vi "Main FPGA 6-axis Servo 2.vi"() -> ()   [LabVIEW 2014]
uses:
  <vilib>/Motion/MotorControl/_s/nism.encoder.config.ctl
  <vilib>/Motion/MotorControl/_s/nism.encoder.incremental.config.ctl
  <vilib>/Motion/MotorControl/_s/nism.incremental.indexCriteria.ctl
  <vilib>/Motion/MotorControl/_s/nism.pid.gains.fxp.18.ctl
  <vilib>/Motion/MotorControl/_s/nism.pi.v.outputRange.fxp.6.12.ctl
  <vilib>/Motion/MotorControl/_s/nism.mdo.splineData.ctl
  <vilib>/Motion/MotorControl/_s/nism.splineInterpolation.type.ctl
  <vilib>/Motion/SoftMotion/Synchronization/nism.softmotionScan.timerConfig.ctl
  <vilib>/Platform/TimedLoop/XDataNode/timing_clust.ctl
  <vilib>/Platform/TimedLoop/XDataNode/nitl_modes.ctl
  <vilib>/Platform/TimedLoop/XDataNode/wakeup.ctl
  <vilib>/Motion/MotorControl/_s/nism.digitalInputs.portA.ctl
  <vilib>/rvi/Emulation/niFpgaGetClockAttributes.vi
  <vilib>/rvi/Emulation/niFpgaSctlEmulationGetInTimedLoop.vi
  <vilib>/rvi/Emulation/niFpgaEmulationReportErrorSimple.vi
  Global FPGA 6-axis.vi
  <vilib>/Motion/MotorControl/_s/nism.interpretControlRegister.indexed.vi
  <vilib>/rvi/Emulation/niFpgaProcessEmulError.vi
  <vilib>/Motion/MotorControl/_s/nism.mdo.read.encoder.vi
  <vilib>/Motion/MotorControl/_s/nism.mdo.read.positionLoopSyncData.vi
  <vilib>/Motion/MotorControl/_s/nism.mdo.read.splineData.vi
  <vilib>/Motion/MotorControl/_s/nism.generateStatusRegister.indexed.vi
  <vilib>/rvi/eio/common/nirviEmuTemplateMethod_errors.vi
  <vilib>/rvi/Emulation/niFpgaCriticalErrorInLSC.vi
  <vilib>/Motion/MotorControl/_s/nism.splineInterpolation.fxp.3.index.vi
  <vilib>/Motion/MotorControl/_s/nism.pid.simple.fxp.index.2.vi
  <vilib>/Motion/MotorControl/_s/nism.mdo.handler.indexed.vi
  <vilib>/Motion/MotorControl/_s/nism.digitalFilter.indexed.vi
  <vilib>/Motion/MotorControl/_s/nism.interpretDIOControl.portA.multiple.vi
  <vilib>/Motion/MotorControl/_s/nism.generateDIOStatus.portA.indexed.2.vi
  <vilib>/Motion/SoftMotion/Synchronization/nism.rioScan.generateSyncScan.vi
  <vilib>/Motion/MotorControl/_s/nism.incremental.p.2.vi
  <vilib>/eio/EIONode/EIONode.xnode
  <vilib>/Platform/TimedLoop/XDataNode/XDataNode.xnode
  <vilib>/Motion/MotorControl/NI_SoftMotion_MotorControlIP.lvlib
  <vilib>/Platform/TimedLoop/XDataNode/XDNodeRunTimeDep.lvlib
  <vilib>/Motion/SoftMotion/Synchronization/NI_SoftMotion_Synchronization.lvlib
panel:
  in  "Reset Encoder 6":bool caption="reset"
  in  "Reset Encoder 5":bool caption="reset"
  in  "Reset Encoder 4":bool caption="reset"
  in  "Reset Encoder 3":bool caption="reset"
  out "position loop sync":T1
  out "spline":T2 {"spline type" items=["cubic b spline", "catmull-rom spline", "linear"]}
  in  "Reset Encoder 2":bool caption="reset"
  out "Velocity Feedback":i16[](array[numeric])
  out "pos. error":i16[](array[numeric])
  out "pos. error exceeded":bool[](array[boolean])
  in  "calls per sample (vel)":u16=2000 caption="calls per sample"
  in  "Limit Ranges":T4[](array[typedef])=[{"output low"=0.0, "output high"=0.0}, {"output low"=0.0, "output high"=0.0}, {"output low"=0.0, "output high"=0.0}, {"output low"=0.0, "output high"=0.0}, {"output low"=0.0, "output high"=0.0}, {"output low"=0.0, "output high"=0.0}]
  in  "Gains":T5[](array[typedef])=[{"kp"=0.0, "kd"=0.0, "ki"=0.0}, {"kp"=0.0, "kd"=0.0, "ki"=0.0}, {"kp"=0.0, "kd"=0.0, "ki"=0.0}, {"kp"=0.0, "kd"=0.0, "ki"=0.0}, {"kp"=0.0, "kd"=0.0, "ki"=0.0}, {"kp"=0.0, "kd"=0.0, "ki"=0.0}]
  out "AO Check":fxp<+/-,20,5>[](array[numeric])
  in  "AO Manual":fxp<+/-,20,5>[](array[numeric])=[0.0, 0.0, 0.0, 0.0, 0.0, 0.0]
  out "Position Feedback":i32[](array[numeric])
  in  "Reset Encoder 1":bool caption="reset"
  out "corrected period":u16
  in  "AO Disabled?":bool
  out "PID loop time (ticks)":u32
  in  "AO Override?":bool
  in  "position error limit":i16=10000
  in  "Encoder filter value (us) Manual":u16=10
  out "encoder config":T6
  out "Home Limits":bool[](array[boolean])
  out "Fwd Limits":bool[](array[boolean])
  out "Rev Limits":bool[](array[boolean])
  out "Drive Enable":bool[](array[boolean])
  in  "Enable value":bool
  in  "Drive Enable override?":bool
  in  "Sync Value":bool
  in  "Sync Enable override?":bool
  out "Sync is Fault":bool
  out "Sync is Locked":bool
  # "Synchronization Loop"
  # "Control Status Loop"
  # "Notes: \n1. This VI provides the communication interface between the NI SoftMotion Engine and the LabVIEW FPGA Module. You must compile this VI for a specific FPGA target before use. After compiling, run the VI before running any of the Express VI examples. For information on moving this example to another FPGA target, refer to ni.com/info and enter info code fpgaex.\n\n2. Only use the Reset Axis button if you are unable to communicate with the axis by any other means. This button resets the device state machine and other VIs to a known state. After resetting the axis, switch the NI Scan Engine from Active Mode to Configuration Mode, then back to Active Mode, before attempting to enable the axis."
  # "(These two buttons \nare for testing\npurposes.)"
  # "(These two buttons \nare for testing\npurposes.)"
  # "Position/PID Loop"
  # "Parameter Check"
  # "AO Debug"
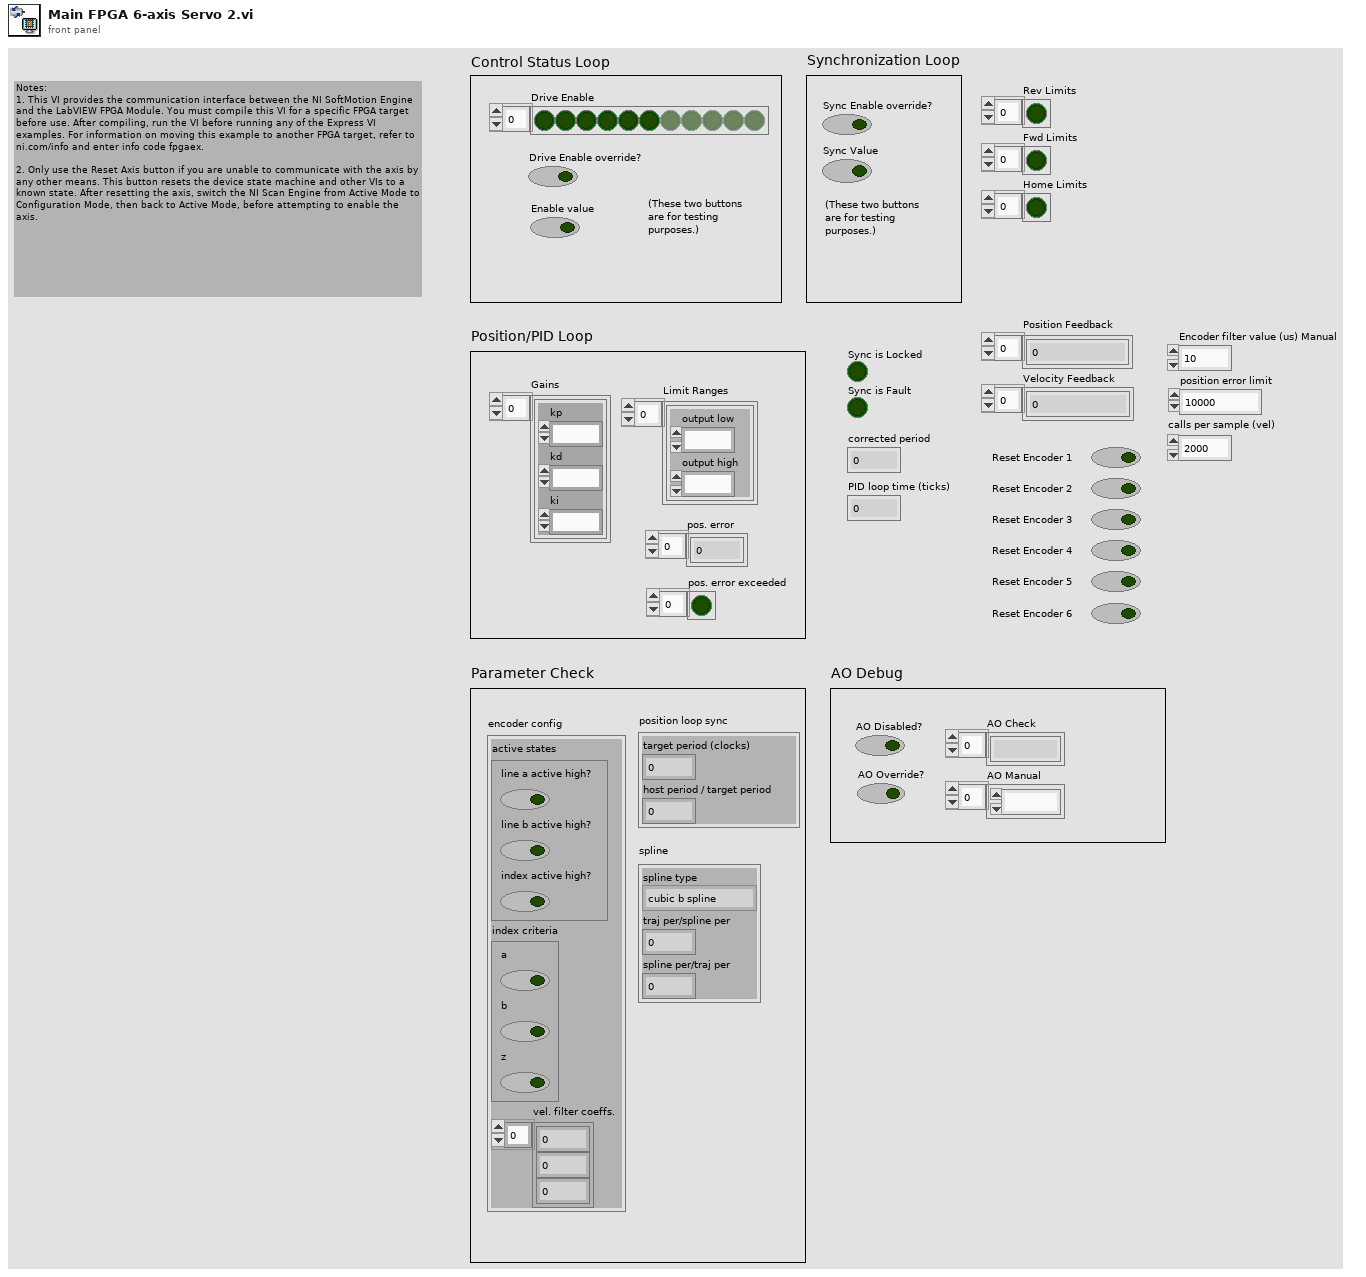
[diagram p1: front panel]
types:
  T1 = typedef "NI_SoftMotion_Synchronization.lvlib/nism.softmotionScan.timerConfig.ctl" = cluster{"target period (clocks)":u16, "host period / target period":u16}
  T2 = typedef "NI_SoftMotion_MotorControlIP.lvlib/nism.mdo.splineData.ctl" = cluster{"spline type":T3, "traj per/spline per":u16, "spline per/traj per":fxp<+,32,0>}
  T3 = typedef "NI_SoftMotion_MotorControlIP.lvlib/nism.splineInterpolation.type.ctl" = u16
  T4 = typedef "NI_SoftMotion_MotorControlIP.lvlib/nism.pi.v.outputRange.fxp.6.12.ctl" = cluster{"output low":fxp<+/-,18,6>, "output high":fxp<+/-,18,6>}
  T5 = typedef "NI_SoftMotion_MotorControlIP.lvlib/nism.pid.gains.fxp.18.ctl" = cluster{"kp":fxp<+,18,7>, "kd":fxp<+,18,7>, "ki":fxp<+,18,0>}
  T6 = typedef "NI_SoftMotion_MotorControlIP.lvlib/nism.encoder.config.ctl" = cluster{"active states":T7, "index criteria":T8, "vel. filter coeffs.":i32[]}
  T7 = typedef "NI_SoftMotion_MotorControlIP.lvlib/nism.encoder.incremental.config.ctl" = cluster{"line a active high?":bool, "line b active high?":bool, "index active high?":bool}
  T8 = typedef "NI_SoftMotion_MotorControlIP.lvlib/nism.incremental.indexCriteria.ctl" = cluster{"a":bool, "b":bool, "z":bool}
  T9 = typedef "XDNodeRunTimeDep.lvlib/timing_clust.ctl" = cluster{"Expected End [f-1]":u64, "Actual End [f-1]":u64, "Finished Late? [f-1]":bool, "Expected End [i-1]":u64, "Actual End [i-1]":u64, "Finished Late? [i-1]":bool, "Expected Start [i]":u64, "Actual Start [i]":u64, "Expected Start [f]":u64, "Actual Start [f]":u64, "Source Name":string, "Structure Name":string, "Period":i64, "Deadline":i64, "Offset":i64, "Start":i64, "Priority":i32, "Timeout":i32, "Mode":T10, "Wakeup Reason":T11, "Error":errorcluster, "Source Type":string, "Secondary Source Type":string, "Global End Time":u64, "Global Start Time":u64, "Frame Duration":u64, "Iteration Duration":u64, "Assigned CPU":i32, "I/O Scan Engine Mode":u32}
  T10 = typedef "XDNodeRunTimeDep.lvlib/nitl_modes.ctl" = enum32{"No Change", "Process missed periods, maintain original phase", "Discard missed periods, maintain original phase", "Process missed periods, ignore original phase", "Discard missed periods, ignore original phase"}
  T11 = typedef "XDNodeRunTimeDep.lvlib/wakeup.ctl" = enum32{"Normal", "Aborted", "Asynchronous wakeup", "Timing source error", "Timed loop error", "Timeout"}
  T12 = typedef "NI_SoftMotion_MotorControlIP.lvlib/nism.digitalInputs.portA.ctl" = cluster{"reverse limit":bool, "forward limit":bool, "home switch":bool, "digital input 0":bool, "digital input 1":bool, "digital input 2":bool, "digital input 3":bool}
  T13 = typedef "NI_SoftMotion_MotorControlIP.lvlib/nism.dio.portA.config.2.ctl" = cluster{"digital filter (us)":u16[], "safe state":T14[]}
  T14 = typedef "nism.safeStates.ctl" = enum8{"Low", "High", "No Change"}
  T15 = typedef "NI_SoftMotion_Synchronization.lvlib/nism.softmotionScan.timerControl.ctl" = cluster{"sm scan":bool, "sm scan count":u32, "sm scan enabled":bool}
  T16 = typedef "NI_SoftMotion_MotorControlIP.lvlib/nism.interpretControlRegister.stateTransition.ctl" = enum8{"Invalid", "Start --> Initializing", "Initializing --> Disabled", "Disabled --> Ready To Switch On", "Ready To Switch On --> Switched On", "Ready To Switch On --> Disable", "Switched On --> Operation Enable", "Switched On --> Ready To Switch On", "Switched On --> Disabled", "Operation Enable --> Switched On", "Operation Enable --> Ready To Switch On", "Operation Enable --> Disabled", "Fault --> Disabled", "Any --> Fault", "None"}
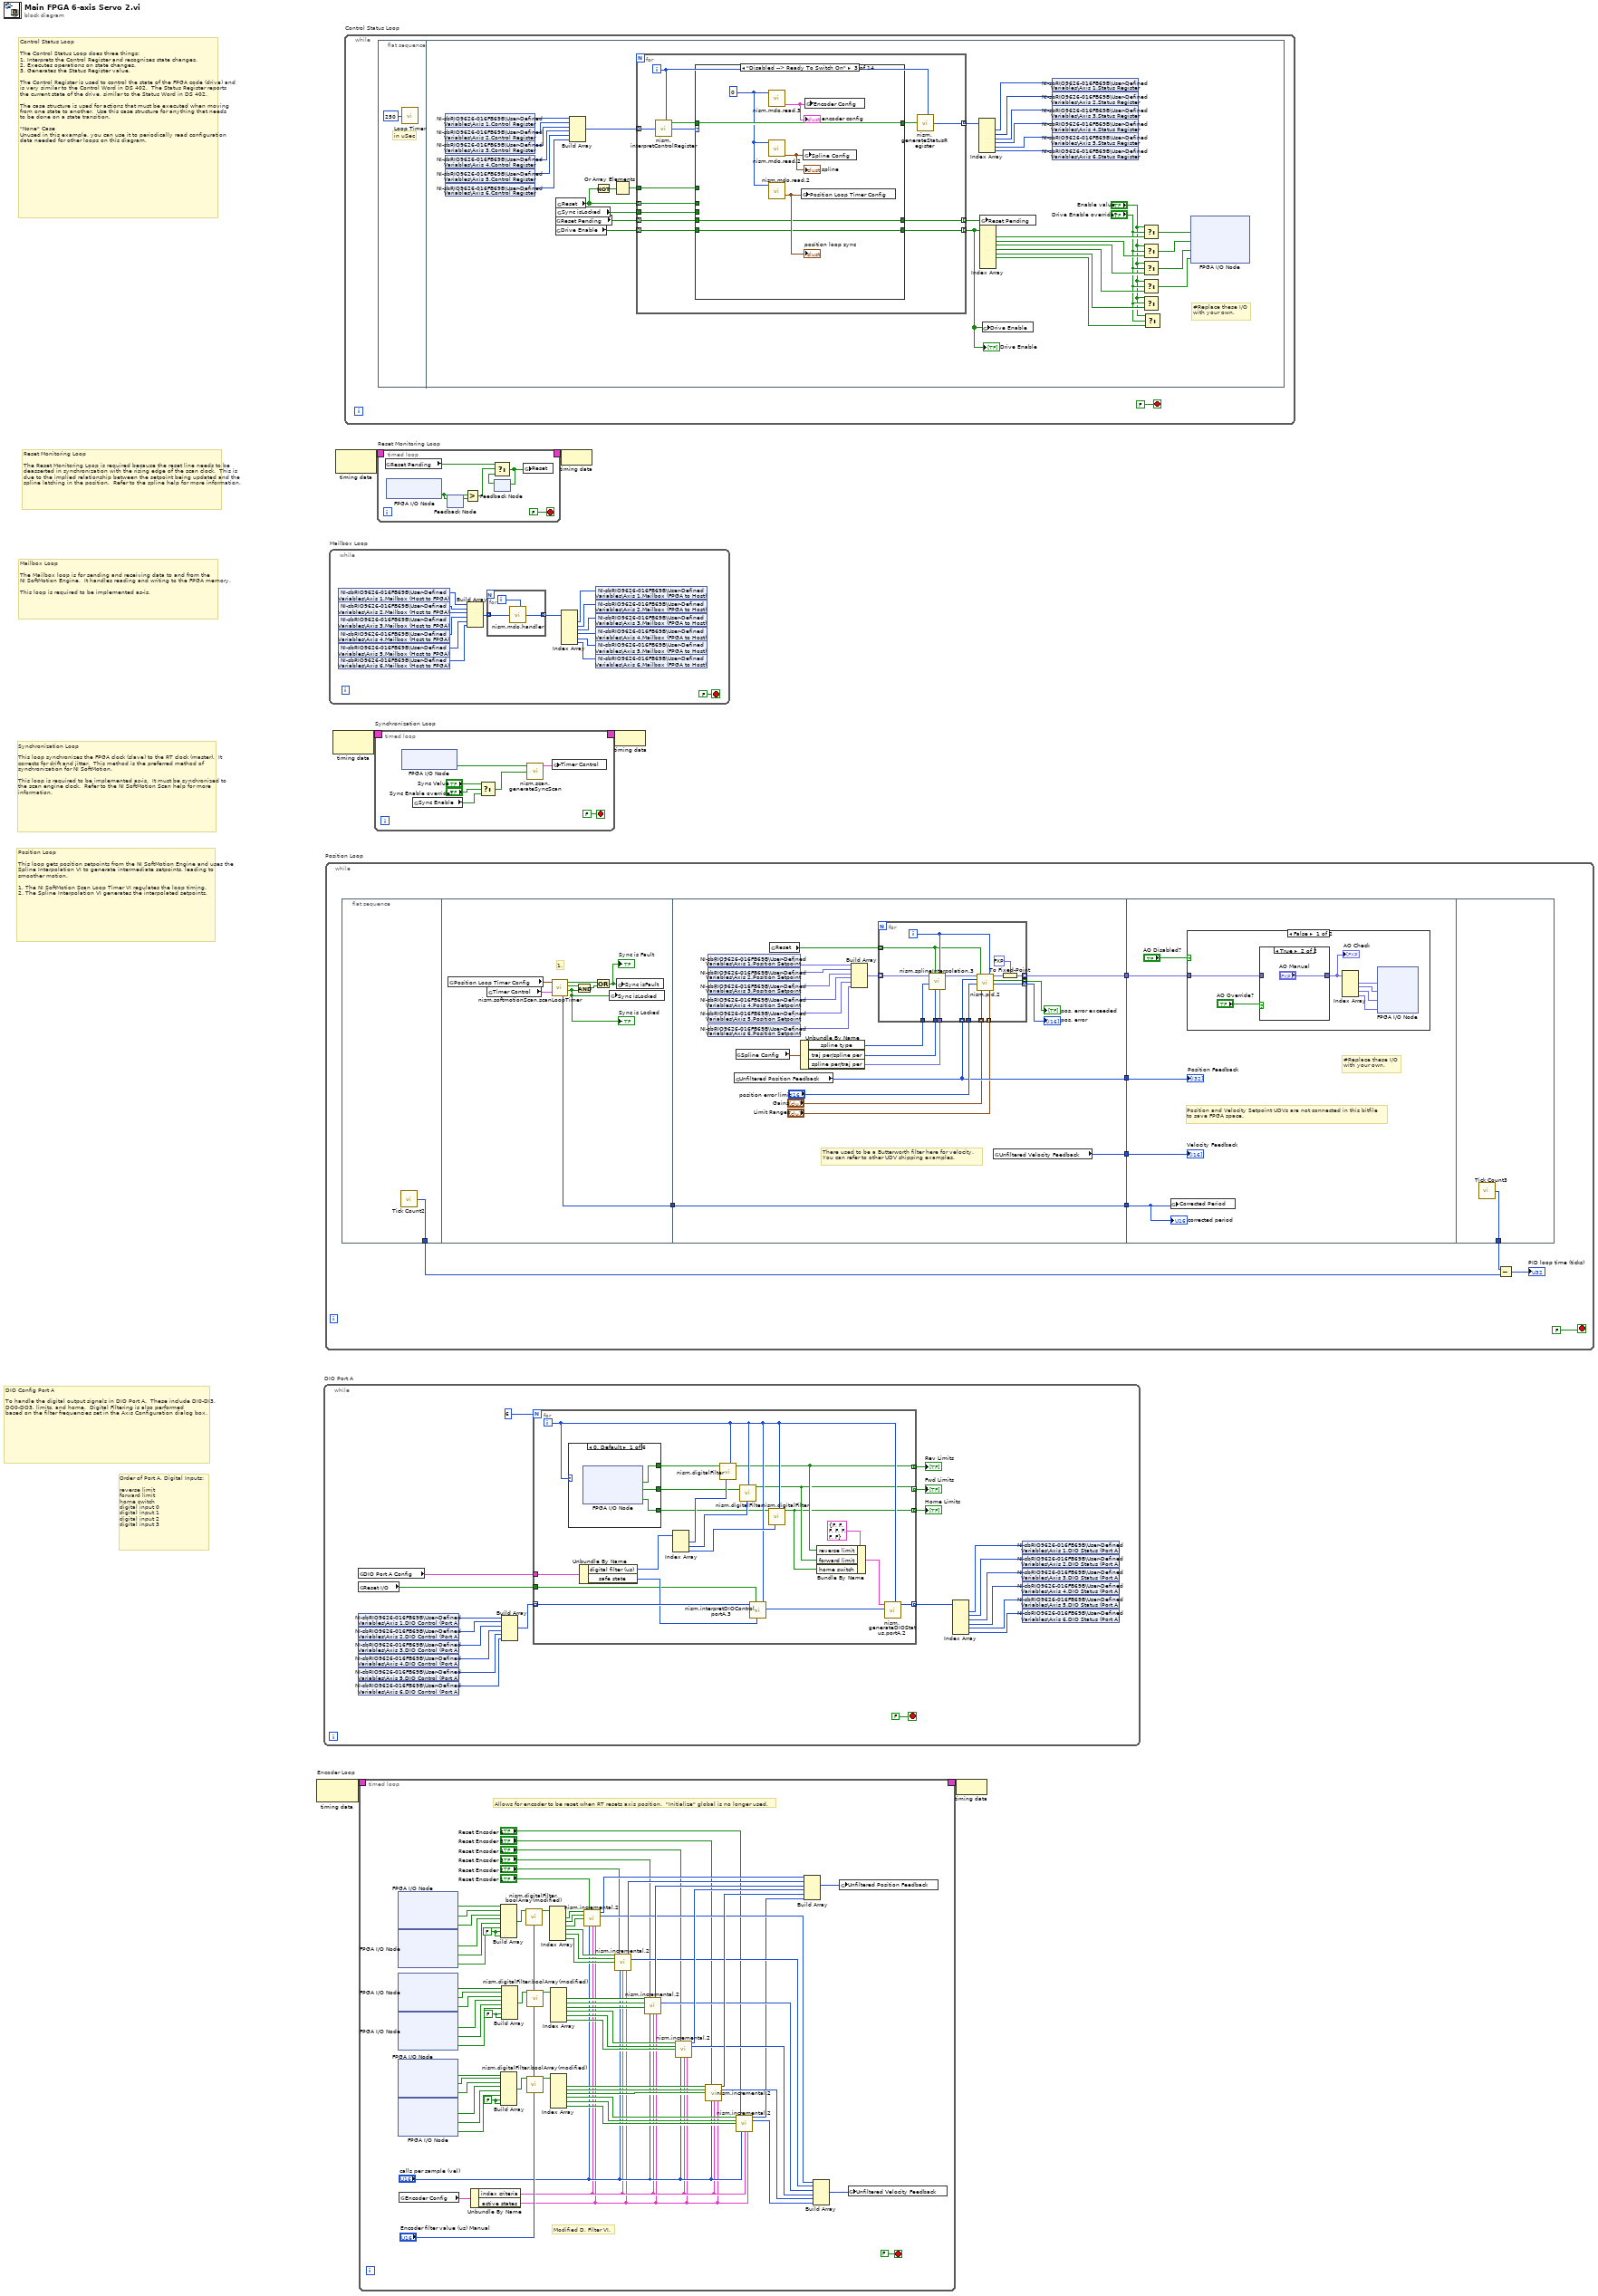
[diagram p0: block diagram]
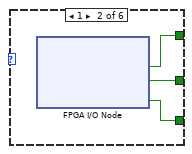
[diagram p2: hidden frame]
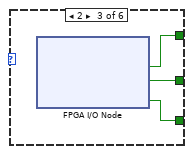
[diagram p3: hidden frame]
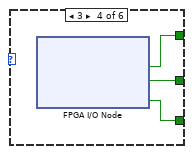
[diagram p4: hidden frame]
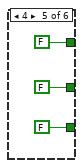
[diagram p5: hidden frame]
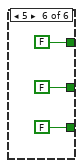
[diagram p6: hidden frame]
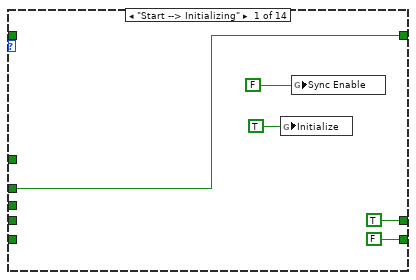
[diagram p9: hidden frame]
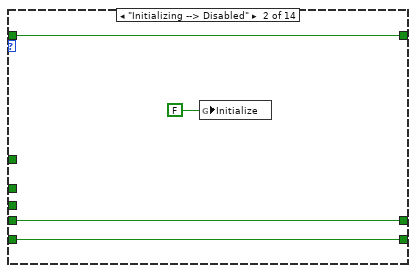
[diagram p10: hidden frame]
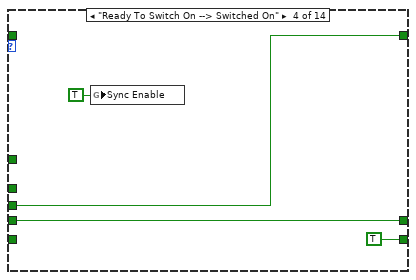
[diagram p11: hidden frame]
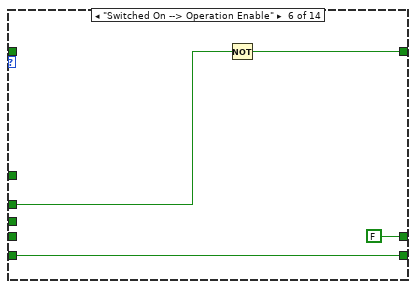
[diagram p13: hidden frame]
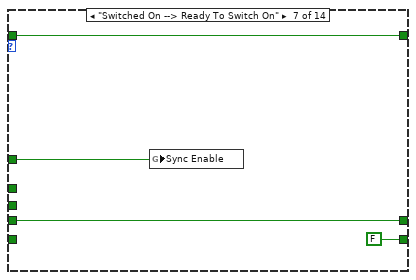
[diagram p14: hidden frame]
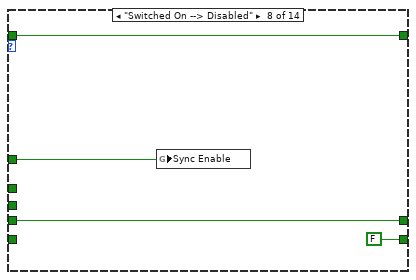
[diagram p15: hidden frame]
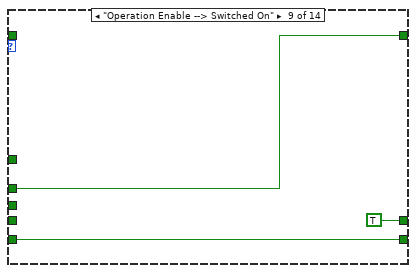
[diagram p16: hidden frame]
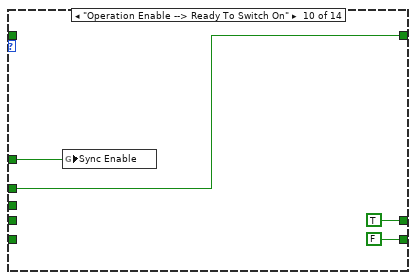
[diagram p17: hidden frame]
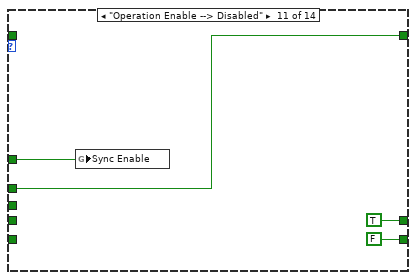
[diagram p18: hidden frame]
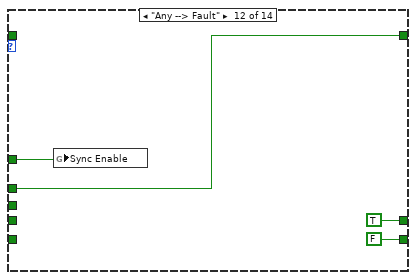
[diagram p19: hidden frame]
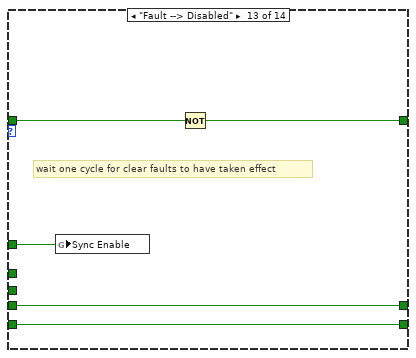
[diagram p20: hidden frame]
diagram:
  # "DIO Config Port A\n\nTo handle the digital output signals in DIO Port A.  These include DI0-DI3, DO0-DO3, limits, and home.  Digital Filtering is also performed\nbased on the filter frequencies set in the Axis Configuration dialog box."
  # "Order of Port A, Digital Inputs:\n\nreverse limit\nforward limit\nhome switch\ndigital input 0\ndigital input 1\ndigital input 2\ndigital input 3"
  # "Position Loop\n\nThis loop gets position setpoints from the NI SoftMotion Engine and uses the Spline Interpolation VI to generate intermediate setpoints, leading to smoother motion.\n\n1. The NI SoftMotion Scan Loop Timer VI regulates the loop timing. \n2. The Spline Interpolation VI generates the interpolated setpoints."
  # "Synchronization Loop\n\nThis loop synchronizes the FPGA clock (slave) to the RT clock (master).  It corrects for drift and jitter.  This method is the preferred method of synchronization for NI SoftMotion.\n\nThis loop is required to be implemented as-is.  It must be synchronized to the scan engine clock.  Refer to the NI SoftMotion Scan help for more information."
  # "Mailbox Loop\n\nThe Mailbox loop is for sending and receiving data to and from the \nNI SoftMotion Engine.  It handles reading and writing to the FPGA memory.\n\nThis loop is required to be implemented as-is."
  # "Reset Monitoring Loop\n\nThe Reset Monitoring Loop is required because the reset line needs to be deasserted in synchronization with the rising edge of the scan clock.  This is due to the implied relationship between the setpoint being updated and the spline latching in the position.  Refer to the spline help for more information."
  # "Control Status Loop\n\nThe Control Status Loop does three things:\n1. Interprets the Control Register and recognizes state changes.\n2. Executes operations on state changes.\n3. Generates the Status Register value.\n\nThe Control Register is used to control the state of the FPGA code (drive) and is very similar to the Control Word in DS 402.  The Status Register reports the current state of the drive, similar to the Status Word in DS 402.\n\nThe case structure is used for actions that must be executed when moving from one state to another.  Use this case structure for anything that needs to be done on a state transition.\n\n\"None\" Case\nUnused in this example, you can use it to periodically read configuration data needed for other loops on this diagram."
  n1 = node-c288() -> (w2:T9)  [unwired: 1 in]
  n2 = while "DIO Port A" {
    stop <- FALSE stop-if-true
    n3 = global read "Global FPGA 6-axis.vi" "DIO Port A Config"() -> (w26:T13)
    n4 = global read "Global FPGA 6-axis.vi" "Reset I/O"() -> (w25:bool)
    n5 = shared-variable "NI-sbRIO9626-016FB69B\\User-Defined Variables\\Axis 1.DIO Control (Port A)"() -> (w23:u32)  [unwired: 1 in, 1 out]
    n6 = shared-variable "NI-sbRIO9626-016FB69B\\User-Defined Variables\\Axis 2.DIO Control (Port A)"() -> (w22:u32)  [unwired: 1 in, 1 out]
    n7 = shared-variable "NI-sbRIO9626-016FB69B\\User-Defined Variables\\Axis 3.DIO Control (Port A)"() -> (w21:u32)  [unwired: 1 in, 1 out]
    n8 = shared-variable "NI-sbRIO9626-016FB69B\\User-Defined Variables\\Axis 4.DIO Control (Port A)"() -> (w20:u32)  [unwired: 1 in, 1 out]
    n9 = shared-variable "NI-sbRIO9626-016FB69B\\User-Defined Variables\\Axis 5.DIO Control (Port A)"() -> (w19:u32)  [unwired: 1 in, 1 out]
    n10 = shared-variable "NI-sbRIO9626-016FB69B\\User-Defined Variables\\Axis 6.DIO Control (Port A)"() -> (w8:u32)  [unwired: 1 in, 1 out]
    n11 = Build Array(w23, w22, w21, w20, w19, w8) -> (w18:u32[])
    n12 = for {
      N: 6 -> [_]
      tunnel: [w45] -> w12 mode=indexing
      tunnel: w18 -> [w44] mode=indexing
      tunnel: w26 -> [w41]
      tunnel: w25 -> [w39]
      tunnel: [w30] -> w11 mode=indexing
      tunnel: [w29] -> w10 mode=indexing
      tunnel: [w28] -> w9 mode=indexing
      i -> [w34]
      n13 = case shown="0, Default" w34 {
        tunnel: [w49 w52 w55 w58 FALSE ("RMC/DIO44") FALSE ("RMC/DIO44")] -> w33
        tunnel: [w47 w50 w53 w56 FALSE ("RMC/DIO61") FALSE ("RMC/DIO61")] -> w32
        tunnel: [w48 w51 w54 w57 FALSE ("RMC/DIO77") FALSE ("RMC/DIO77")] -> w31
        frame 0, Default {
          n14 = xnode "FPGA I/O Node"() -> ("RMC/DIO29"=w49:bool, "RMC/DIO93"=w48:bool, "RMC/DIO11"=w47:bool)  [unwired: 3 in, 3 out]
        }
        frame 1 {
          n15 = xnode "FPGA I/O Node"() -> ("RMC/DIO44"=w52:bool, "RMC/DIO77"=w51:bool, "RMC/DIO61"=w50:bool)  [unwired: 3 in, 3 out]
        }
        frame 2 {
          n16 = xnode "FPGA I/O Node"() -> ("RMC/DIO31"=w55:bool, "RMC/DIO95"=w54:bool, "RMC/DIO13"=w53:bool)  [unwired: 3 in, 3 out]
        }
        frame 3 {
          n17 = xnode "FPGA I/O Node"() -> ("RMC/DIO47"=w58:bool, "RMC/DIO46"=w57:bool, "RMC/DIO79"=w56:bool)  [unwired: 3 in, 3 out]
        }
        frame 4 {
        }
        frame 5 {
        }
      }
      n18 = Unbundle By Name(w41) -> ("digital filter (us)"=w35:u16[], "safe state"=w40:T14[])
      n19 = Index Array(array=w35) -> (element #1=w36:u16, element #2=w37:u16, element #3=w38:u16)  [unwired: 3 in]
      n20 = call-poly <vilib>:"nism.digitalFilter.vi"("index"=w34, "filter value (us)"=w36, "input signal"=w33) -> ("output signal"=w30:bool)  [unwired: 8 in]
      n21 = call-poly <vilib>:"nism.digitalFilter.vi"("index"=w34, "filter value (us)"=w37, "input signal"=w31) -> ("output signal"=w29:bool)  [unwired: 8 in]
      n22 = call-poly <vilib>:"nism.interpretDIOControl.portA.3.vi"("index"=w34, "safe state"=w40, "reset"=w39, "dio control(port a)"=w44) -> ("reset latches"=w46:u8)  [unwired: 6 in, 1 out]
      n23 = call-poly <vilib>:"nism.digitalFilter.vi"("index"=w34, "filter value (us)"=w38, "input signal"=w32) -> ("output signal"=w28:bool)  [unwired: 8 in]
      n24 = Bundle By Name(cluster=T12 {"reverse limit"=FALSE, "forward limit"=FALSE, "home switch"=FALSE, "digital input 0"=FALSE, "digital input 1"=FALSE, "digital input 2"=FALSE, "digital input 3"=FALSE} ("$(driveInterface.digitalInputs.shortName)"), "reverse limit"=w30, "forward limit"=w29, "home switch"=w28) -> (w42:T12)
      n25 = call-poly <vilib>:"nism.generateDIOStatus.portA.2.vi"("index"=w34, "reset latches"=w46, "digital inputs"=w42) -> ("dio status(port a)"=w45:u32)  [unwired: 8 in]
    }
    "Rev Limits" <- w11
    "Fwd Limits" <- w10
    "Home Limits" <- w9
    n26 = Index Array(array=w12) -> (element #1=w17:u32, element #2=w16:u32, element #3=w15:u32, element #4=w14:u32, element #5=w13:u32, element #6=w7:u32)  [unwired: 6 in]
    n27 = shared-variable "NI-sbRIO9626-016FB69B\\User-Defined Variables\\Axis 1.DIO Status (Port A)"(w17) -> ()  [unwired: 1 in, 1 out]
    n28 = shared-variable "NI-sbRIO9626-016FB69B\\User-Defined Variables\\Axis 2.DIO Status (Port A)"(w16) -> ()  [unwired: 1 in, 1 out]
    n29 = shared-variable "NI-sbRIO9626-016FB69B\\User-Defined Variables\\Axis 3.DIO Status (Port A)"(w15) -> ()  [unwired: 1 in, 1 out]
    n30 = shared-variable "NI-sbRIO9626-016FB69B\\User-Defined Variables\\Axis 4.DIO Status (Port A)"(w14) -> ()  [unwired: 1 in, 1 out]
    n31 = shared-variable "NI-sbRIO9626-016FB69B\\User-Defined Variables\\Axis 5.DIO Status (Port A)"(w13) -> ()  [unwired: 1 in, 1 out]
    n32 = shared-variable "NI-sbRIO9626-016FB69B\\User-Defined Variables\\Axis 6.DIO Status (Port A)"(w7) -> ()  [unwired: 1 in, 1 out]
  }
  n33 = while "Position Loop" {
    stop <- FALSE stop-if-true
    n34 = flat-sequence {
      tunnel: [w74] -> w68
      tunnel: [w75] -> w71
      tunnel: [w99] -> w72
      tunnel: w71 -> [w99]
      tunnel: [w89] -> w70
      tunnel: [w93] -> w66
      tunnel: [w83] -> w65
      tunnel: w72 -> [w124]
      tunnel: w70 -> [w120]
      tunnel: w66 -> [w123]
      tunnel: w65 -> [w121]
      tunnel: [w134] -> w69
      frame #0 {
        n35 = call "Tick Count2"() -> ("Tick Count(Ticks)"=w74:u32)
      }
      frame #1 {
        # "1."
        n36 = global read "Global FPGA 6-axis.vi" "Position Loop Timer Config"() -> (w77:T1)
        n37 = global read "Global FPGA 6-axis.vi" "Timer Control"() -> (w76:T15)
        n38 = call <vilib>:"nism.softmotionScan.scanLoopTimer.vi"("timer control"=w76, "timer config"=w77) -> ("scan running?"=w79:bool, "finished late?"=w81:bool, "fault occurred?"=w82:bool, "corrected period"=w75:u16)  [unwired: 5 in, 1 out]
        "Sync is Locked" <- w79
        n39 = Compound Arithmetic op=AND(w81, w79) -> (w80:bool)
        n40 = Compound Arithmetic op=OR(w82, w80) -> (w78:bool)
        "Sync is Fault" <- w78
        n41 = global write "Global FPGA 6-axis.vi" "Sync isLocked"(w79) -> ()
        n42 = global write "Global FPGA 6-axis.vi" "Sync isFault"(w78) -> ()
      }
      frame #2 {
        # "There used to be a Butterworth filter here for velocity.  \nYou can refer to other UDV shipping examples."
        n43 = shared-variable "NI-sbRIO9626-016FB69B\\User-Defined Variables\\Axis 1.Position Setpoint"() -> (w94:fxp<+/-,64,32>)  [unwired: 1 in, 1 out]
        n44 = shared-variable "NI-sbRIO9626-016FB69B\\User-Defined Variables\\Axis 2.Position Setpoint"() -> (w98:fxp<+/-,64,32>)  [unwired: 1 in, 1 out]
        n45 = shared-variable "NI-sbRIO9626-016FB69B\\User-Defined Variables\\Axis 3.Position Setpoint"() -> (w97:fxp<+/-,64,32>)  [unwired: 1 in, 1 out]
        n46 = shared-variable "NI-sbRIO9626-016FB69B\\User-Defined Variables\\Axis 4.Position Setpoint"() -> (w96:fxp<+/-,64,32>)  [unwired: 1 in, 1 out]
        n47 = shared-variable "NI-sbRIO9626-016FB69B\\User-Defined Variables\\Axis 5.Position Setpoint"() -> (w95:fxp<+/-,64,32>)  [unwired: 1 in, 1 out]
        n48 = shared-variable "NI-sbRIO9626-016FB69B\\User-Defined Variables\\Axis 6.Position Setpoint"() -> (w86:fxp<+/-,64,32>)  [unwired: 1 in, 1 out]
        n49 = global read "Global FPGA 6-axis.vi" "Unfiltered Position Feedback"() -> (w89:i32[])
        n50 = global read "Global FPGA 6-axis.vi" "Spline Config"() -> (w100:T2)
        n51 = global read "Global FPGA 6-axis.vi" "Reset"() -> (w91:bool[])
        n52 = Unbundle By Name(w100) -> ("spline type"=w103:T3, "traj per/spline per"=w102:u16, "spline per/traj per"=w101:fxp<+,32,0>)
        n53 = Build Array(w94, w98, w97, w96, w95, w86) -> (w92:fxp<+/-,64,32>[])
        n54 = for {
          tunnel: w103 -> [w119]
          tunnel: w102 -> [w118]
          tunnel: w101 -> [w117]
          tunnel: "Limit Ranges" -> [w115] mode=indexing
          tunnel: [w105] -> w93 mode=indexing
          tunnel: w92 -> [w114] mode=indexing
          tunnel: w91 -> [w112] mode=indexing
          tunnel: w89 -> [w111] mode=indexing
          tunnel: "position error limit" -> [w110]
          tunnel: [w109] -> w85 mode=indexing
          tunnel: [w108] -> w84 mode=indexing
          tunnel: "Gains" -> [w104] mode=indexing
          i -> [w113]
          n55 = call-poly <vilib>:"nism.splineInterpolation.3.vi"("1 / calls per sample"=w117, "index"=w113, "calls per sample"=w118, "reset"=w112, "spline type"=w119, "x"=w114) -> ("xi"=w116:fxp<+/-,64,32>)  [unwired: 4 in, 1 out]
          n56 = call-poly <vilib>:"nism.pid.2.vi"("position setpoint"=w116, "position feedback"=w111, "position error limit"=w110, "reset"=w112, "gains"=w104, "index"=w113, "output range"=w115) -> ("current setpoint"=w106:fxp<+/-,18,6>, "pos. error exceeded"=w109:bool, "position error"=w108:i16)  [unwired: 10 in]
          n57 = To Fixed-Point(fixed-point type=fxp<+/-,20,5> 0.0 ("AO 1"), number=w106) -> (fixed-point=w105:fxp<+/-,20,5>)
        }
        "pos. error exceeded" <- w85
        "pos. error" <- w84
        n58 = global read "Global FPGA 6-axis.vi" "Unfiltered Velocity Feedback"() -> (w83:i16[])
      }
      frame #3 {
        # "Position and Velocity Setpoint UDVs are not connected in this bitfile\nto save FPGA space."
        # "#Replace these I/O\nwith your own."
        n59 = global write "Global FPGA 6-axis.vi" "Corrected Period"(w124) -> ()
        n60 = case shown="False" "AO Disabled?" {
          tunnel: w123 -> [w130 _]
          frame False {
            n61 = case shown="True" "AO Override?" {
              tunnel: w130 -> [w132 _]
              tunnel: [w132 "AO Manual"] -> w129
              frame False {
              }
              frame True {
              }
            }
            "AO Check" <- w129
            n62 = Index Array(array=w129) -> (element #1=w128:fxp<+/-,20,5>, element #2=w127:fxp<+/-,20,5>, element #3=w126:fxp<+/-,20,5>, element #4=w125:fxp<+/-,20,5>)  [unwired: 4 in]
            n63 = xnode "FPGA I/O Node"("AO0"=w128, "AO1"=w127, "AO2"=w126, "AO3"=w125) -> ()  [unwired: 4 in, 4 out]
          }
          frame True {
          }
        }
        "corrected period" <- w124
        "Position Feedback" <- w120
        "Velocity Feedback" <- w121
      }
      frame #4 {
        n64 = call "Tick Count3"() -> ("Tick Count(Ticks)"=w134:u32)
      }
    }
    n65 = Subtract(x=w69, y=w68) -> (x-y=→"PID loop time (ticks)":u32)
  }
  n66 = while "Mailbox Loop" {
    stop <- FALSE stop-if-true
    n67 = shared-variable "NI-sbRIO9626-016FB69B\\User-Defined Variables\\Axis 1.Mailbox (Host to FPGA)"() -> (w146:u64)  [unwired: 1 in, 1 out]
    n68 = shared-variable "NI-sbRIO9626-016FB69B\\User-Defined Variables\\Axis 2.Mailbox (Host to FPGA)"() -> (w145:u64)  [unwired: 1 in, 1 out]
    n69 = shared-variable "NI-sbRIO9626-016FB69B\\User-Defined Variables\\Axis 3.Mailbox (Host to FPGA)"() -> (w144:u64)  [unwired: 1 in, 1 out]
    n70 = shared-variable "NI-sbRIO9626-016FB69B\\User-Defined Variables\\Axis 4.Mailbox (Host to FPGA)"() -> (w143:u64)  [unwired: 1 in, 1 out]
    n71 = shared-variable "NI-sbRIO9626-016FB69B\\User-Defined Variables\\Axis 5.Mailbox (Host to FPGA)"() -> (w142:u64)  [unwired: 1 in, 1 out]
    n72 = shared-variable "NI-sbRIO9626-016FB69B\\User-Defined Variables\\Axis 6.Mailbox (Host to FPGA)"() -> (w135:u64)  [unwired: 1 in, 1 out]
    n73 = Build Array(w146, w145, w144, w143, w142, w135) -> (w148:u64[])
    n74 = for {
      tunnel: w148 -> [w152] mode=indexing
      tunnel: [w151] -> w147 mode=indexing
      i -> [w150]
      n75 = call-poly <vilib>:"nism.mdo.handler.vi"("mbox (host to fpga)"=w152, "axis index"=w150) -> ("mbox (fpga to host)"=w151:u64)  [unwired: 7 in]
    }
    n76 = Index Array(array=w147) -> (element #1=w141:u64, element #2=w140:u64, element #3=w139:u64, element #4=w138:u64, element #5=w137:u64, element #6=w136:u64)  [unwired: 6 in]
    n77 = shared-variable "NI-sbRIO9626-016FB69B\\User-Defined Variables\\Axis 1.Mailbox (FPGA to Host)"(w141) -> ()  [unwired: 1 in, 1 out]
    n78 = shared-variable "NI-sbRIO9626-016FB69B\\User-Defined Variables\\Axis 2.Mailbox (FPGA to Host)"(w140) -> ()  [unwired: 1 in, 1 out]
    n79 = shared-variable "NI-sbRIO9626-016FB69B\\User-Defined Variables\\Axis 3.Mailbox (FPGA to Host)"(w139) -> ()  [unwired: 1 in, 1 out]
    n80 = shared-variable "NI-sbRIO9626-016FB69B\\User-Defined Variables\\Axis 4.Mailbox (FPGA to Host)"(w138) -> ()  [unwired: 1 in, 1 out]
    n81 = shared-variable "NI-sbRIO9626-016FB69B\\User-Defined Variables\\Axis 5.Mailbox (FPGA to Host)"(w137) -> ()  [unwired: 1 in, 1 out]
    n82 = shared-variable "NI-sbRIO9626-016FB69B\\User-Defined Variables\\Axis 6.Mailbox (FPGA to Host)"(w136) -> ()  [unwired: 1 in, 1 out]
  }
  n83 = node-c288() -> (w6:T9)  [unwired: 1 in]
  n84 = node-c288() -> (w4:T9)  [unwired: 1 in]
  n85 = while "Control Status Loop" {
    stop <- FALSE stop-if-true
    n86 = flat-sequence {
      frame #0 {
        # "in uSec"
        n87 = call "Loop Timer"("Count(uSec)"=u32 250) -> ()  [unwired: 1 out]
      }
      frame #1 {
        # "#Replace these I/O\nwith your own."
        n88 = shared-variable "NI-sbRIO9626-016FB69B\\User-Defined Variables\\Axis 1.Control Register"() -> (w178:u32)  [unwired: 1 in, 1 out]
        n89 = shared-variable "NI-sbRIO9626-016FB69B\\User-Defined Variables\\Axis 2.Control Register"() -> (w177:u32)  [unwired: 1 in, 1 out]
        n90 = shared-variable "NI-sbRIO9626-016FB69B\\User-Defined Variables\\Axis 3.Control Register"() -> (w176:u32)  [unwired: 1 in, 1 out]
        n91 = shared-variable "NI-sbRIO9626-016FB69B\\User-Defined Variables\\Axis 4.Control Register"() -> (w175:u32)  [unwired: 1 in, 1 out]
        n92 = shared-variable "NI-sbRIO9626-016FB69B\\User-Defined Variables\\Axis 5.Control Register"() -> (w174:u32)  [unwired: 1 in, 1 out]
        n93 = shared-variable "NI-sbRIO9626-016FB69B\\User-Defined Variables\\Axis 6.Control Register"() -> (w159:u32)  [unwired: 1 in, 1 out]
        n94 = global read "Global FPGA 6-axis.vi" "Reset Pending"() -> (w182:bool[])
        n95 = global read "Global FPGA 6-axis.vi" "Drive Enable"() -> (w181:bool[])
        n96 = global read "Global FPGA 6-axis.vi" "Reset"() -> (w183:bool[])
        n97 = global read "Global FPGA 6-axis.vi" "Sync isLocked"() -> (w188:bool)
        n98 = Build Array(w178, w177, w176, w175, w174, w159) -> (w187:u32[])
        n99 = Not(x=w183) -> (.not. x?=w185:bool[])
        n100 = Or Array Elements(Boolean array=w185) -> (logical OR=w184:bool)
        n101 = for {
          tunnel: w183 -> [w197] mode=indexing
          tunnel: w188 -> [w196]
          tunnel: w187 -> [w198] mode=indexing
          tunnel: [w195] -> w179 mode=indexing
          tunnel: [w194] -> w186 mode=indexing
          tunnel: [w193] -> w180 mode=indexing
          tunnel: w184 -> [w192]
          tunnel: w182 -> [w191] mode=indexing
          tunnel: w181 -> [w190] mode=indexing
          i -> [w199]
          n102 = call-poly <vilib>:"nism.interpretControlRegister.vi"("control register"=w198, "axis index"=w199) -> ("transition occurred"=w200:bool, "state transition"=w189:T16)  [unwired: 6 in]
          n103 = case shown="\"Disabled --> Ready To Switch On\"" w189 {
            tunnel: w200 -> [_ w210 w217 _ w224 _ w232 w236 _ _ _ _ w256 _]
            tunnel: [w206 w210 w217 w219 w224 w228 w232 w236 w238 w241 w245 w249 w255 _] -> w201
            tunnel: w197 -> [w206 _ _ _ _ w227 _ _ w238 w241 w245 w249 _ _]
            tunnel: w196 -> [_ _ _ w219 _ _ _ _ _ _ _ _ _ _]
            tunnel: [TRUE ("Write.Reset Pending") w209 w214 w218 w223 FALSE ("Write.Reset Pending") w229 w233 TRUE ("Write.Reset Pending") TRUE ("Write.Reset Pending") TRUE ("Write.Reset Pending") TRUE ("Write.Reset Pending") w253 w258] -> w194
            tunnel: [FALSE ("Write.Drive Enable") w208 w213 TRUE ("Write.Drive Enable") w222 w225 FALSE ("Write.Drive Enable") FALSE ("Write.Drive Enable") w237 FALSE ("Write.Drive Enable") FALSE ("Write.Drive Enable") FALSE ("Write.Drive Enable") w252 w257] -> w193
            tunnel: w192 -> [_ _ _ _ _ _ w230 w234 _ w240 w244 w248 w254 _]
            tunnel: w191 -> [_ w209 w214 w218 w223 _ w229 w233 _ _ _ _ w253 w258]
            tunnel: w190 -> [_ w208 w213 _ w222 w225 _ _ w237 _ _ _ w252 w257]
            frame "Start --> Initializing" {
              n104 = global write "Global FPGA 6-axis.vi" "Initialize"(TRUE ("Initialize")) -> ()
              n105 = global write "Global FPGA 6-axis.vi" "Sync Enable"(FALSE ("Sync Enable")) -> ()
            }
            frame "Initializing --> Disabled" {
              n106 = global write "Global FPGA 6-axis.vi" "Initialize"(FALSE ("Initialize")) -> ()
            }
            frame "Disabled --> Ready To Switch On" {
              w211 = 0 ("axis index")
              n107 = call-poly <vilib>:"nism.mdo.read.3.vi"("axis index"=w211) -> ("encoder config"=w212:T6)  [unwired: 10 in]
              "encoder config" <- w212
              n108 = call-poly <vilib>:"nism.mdo.read.2.vi"("axis index"=w211) -> ("spline"=w216:T2)  [unwired: 10 in]
              "spline" <- w216
              n109 = call-poly <vilib>:"nism.mdo.read.2.vi"("axis index"=w211) -> ("position loop sync"=w215:T1)  [unwired: 10 in]
              "position loop sync" <- w215
              n110 = global write "Global FPGA 6-axis.vi" "Position Loop Timer Config"(w215) -> ()
              n111 = global write "Global FPGA 6-axis.vi" "Spline Config"(w216) -> ()
              n112 = global write "Global FPGA 6-axis.vi" "Encoder Config"(w212) -> ()
            }
            frame "Ready To Switch On --> Switched On" {
              n113 = global write "Global FPGA 6-axis.vi" "Sync Enable"(TRUE ("Sync Enable")) -> ()
            }
            frame "Ready To Switch On --> Disable" {
            }
            frame "Switched On --> Operation Enable" {
              n114 = Not(x=w227) -> (.not. x?=w228:bool)
            }
            frame "Switched On --> Ready To Switch On" {
              n115 = global write "Global FPGA 6-axis.vi" "Sync Enable"(w230) -> ()
            }
            frame "Switched On --> Disabled" {
              n116 = global write "Global FPGA 6-axis.vi" "Sync Enable"(w234) -> ()
            }
            frame "Operation Enable --> Switched On" {
            }
            frame "Operation Enable --> Ready To Switch On" {
              n117 = global write "Global FPGA 6-axis.vi" "Sync Enable"(w240) -> ()
            }
            frame "Operation Enable --> Disabled" {
              n118 = global write "Global FPGA 6-axis.vi" "Sync Enable"(w244) -> ()
            }
            frame "Any --> Fault" {
              n119 = global write "Global FPGA 6-axis.vi" "Sync Enable"(w248) -> ()
            }
            frame "Fault --> Disabled" {
              # "wait one cycle for clear faults to have taken effect"
              n120 = global write "Global FPGA 6-axis.vi" "Sync Enable"(w254) -> ()
              n121 = Not(x=w256) -> (.not. x?=w255:bool)
            }
            frame "None", Default {
            }
          }
          n122 = call-poly <vilib>:"nism.generateStatusRegister.vi"("transition success"=w201, "axis index"=w199) -> ("status register"=w195:u32)  [unwired: 7 in]
        }
        "Drive Enable" <- w180
        n123 = Index Array(array=w179) -> (element #1=w173:u32, element #2=w172:u32, element #3=w171:u32, element #4=w170:u32, element #5=w169:u32, element #6=w158:u32)  [unwired: 6 in]
        n124 = global write "Global FPGA 6-axis.vi" "Reset Pending"(w186) -> ()
        n125 = Index Array(array=w180) -> (element #1=w168:bool, element #2=w167:bool, element #3=w166:bool, element #4=w165:bool, element #5=w164:bool, element #6=w157:bool)  [unwired: 8 in, 2 out]
        n126 = global write "Global FPGA 6-axis.vi" "Drive Enable"(w180) -> ()
        n127 = shared-variable "NI-sbRIO9626-016FB69B\\User-Defined Variables\\Axis 1.Status Register"(w173) -> ()  [unwired: 1 in, 1 out]
        n128 = shared-variable "NI-sbRIO9626-016FB69B\\User-Defined Variables\\Axis 2.Status Register"(w172) -> ()  [unwired: 1 in, 1 out]
        n129 = shared-variable "NI-sbRIO9626-016FB69B\\User-Defined Variables\\Axis 3.Status Register"(w171) -> ()  [unwired: 1 in, 1 out]
        n130 = shared-variable "NI-sbRIO9626-016FB69B\\User-Defined Variables\\Axis 4.Status Register"(w170) -> ()  [unwired: 1 in, 1 out]
        n131 = shared-variable "NI-sbRIO9626-016FB69B\\User-Defined Variables\\Axis 5.Status Register"(w169) -> ()  [unwired: 1 in, 1 out]
        n132 = shared-variable "NI-sbRIO9626-016FB69B\\User-Defined Variables\\Axis 6.Status Register"(w158) -> ()  [unwired: 1 in, 1 out]
        n133 = Select(t="Enable value", s="Drive Enable override?", f=w168) -> (s? t:f=w163:bool)
        n134 = Select(t="Enable value", s="Drive Enable override?", f=w167) -> (s? t:f=w162:bool)
        n135 = Select(t="Enable value", s="Drive Enable override?", f=w166) -> (s? t:f=w161:bool)
        n136 = Select(t="Enable value", s="Drive Enable override?", f=w165) -> (s? t:f=w160:bool)
        n137 = Select(t="Enable value", s="Drive Enable override?", f=w164) -> ()  [unwired: 1 out]
        n138 = Select(t="Enable value", s="Drive Enable override?", f=w157) -> ()  [unwired: 1 out]
        n139 = xnode "FPGA I/O Node"("RMC/DIO28"=w163, "RMC/DIO12"=w162, "RMC/DIO30"=w161, "RMC/DIO14"=w160) -> ()  [unwired: 4 in, 4 out]
      }
    }
  }
  n140 = timed-loop "Encoder Loop" {
    timing: w2 -> [_]
    timing-out: [_] -> w1
    stop <- FALSE stop-if-true
    w286 = FALSE ("element")
    w287 = FALSE ("element")
    w303 = FALSE ("element")
    # "Allows for encoder to be reset when RT resets axis position.  \"Initialize\" global is no longer used."
    # "Modified D. Filter VI."
    n141 = xnode "FPGA I/O Node"() -> ("RMC/DIO60"=w327:bool, "RMC/DIO42"=w328:bool, "RMC/DIO75"=w326:bool)  [unwired: 3 in, 3 out]
    n142 = xnode "FPGA I/O Node"() -> ("RMC/DIO59"=w308:bool, "RMC/DIO92"=w307:bool, "RMC/DIO10"=w306:bool)  [unwired: 3 in, 3 out]
    n143 = xnode "FPGA I/O Node"() -> ("RMC/DIO74"=w299:bool, "RMC/DIO27"=w298:bool, "RMC/DIO91"=w297:bool)  [unwired: 3 in, 3 out]
    n144 = xnode "FPGA I/O Node"() -> ("RMC/DIO9"=w296:bool, "RMC/DIO41"=w295:bool, "RMC/DIO26"=w294:bool)  [unwired: 3 in, 3 out]
    n145 = xnode "FPGA I/O Node"() -> ("RMC/DIO58"=w280:bool, "RMC/DIO40"=w281:bool, "RMC/DIO73"=w282:bool)  [unwired: 3 in, 3 out]
    n146 = xnode "FPGA I/O Node"() -> ("RMC/DIO57"=w283:bool, "RMC/DIO90"=w284:bool, "RMC/DIO8"=w285:bool)  [unwired: 3 in, 3 out]
    n147 = global read "Global FPGA 6-axis.vi" "Encoder Config"() -> (w263:T6)
    n148 = Unbundle By Name(w263) -> ("index criteria"=w266:T8, "active states"=w265:T7)
    n149 = Build Array(w327, w328, w326, w308, w307, w306, w303, w303) -> (w325:bool[])
    n150 = Build Array(w280, w281, w282, w283, w284, w285, w286, w286) -> (w279:bool[])
    n151 = Build Array(w299, w298, w297, w296, w295, w294, w287, w287) -> (w304:bool[])
    n152 = call "nism.digitalFilter.boolArray(modified).vi"("filter value (us)"="Encoder filter value (us) Manual", "input signal"=w325) -> ("output signal"=w324:bool[])  [unwired: 9 in]
    n153 = call "nism.digitalFilter.boolArray(modified).vi"("filter value (us)"="Encoder filter value (us) Manual", "input signal"=w279) -> ("output signal"=w278:bool[])  [unwired: 9 in]
    n154 = call "nism.digitalFilter.boolArray(modified).vi"("filter value (us)"="Encoder filter value (us) Manual", "input signal"=w304) -> ("output signal"=w305:bool[])  [unwired: 9 in]
    n155 = Index Array(array=w324) -> (element #1=w323:bool, element #2=w322:bool, element #3=w321:bool, element #4=w302:bool, element #5=w301:bool, element #6=w300:bool)  [unwired: 6 in]
    n156 = Index Array(array=w278) -> (element #1=w277:bool, element #2=w276:bool, element #3=w275:bool, element #4=w272:bool, element #5=w271:bool, element #6=w270:bool)  [unwired: 6 in]
    n157 = Index Array(array=w305) -> (element #1=w293:bool, element #2=w292:bool, element #3=w291:bool, element #4=w290:bool, element #5=w289:bool, element #6=w288:bool)  [unwired: 6 in]
    n158 = call-poly <vilib>:"nism.incremental.2.vi"("a phase"=w323, "reset"="Reset Encoder 1", "b phase"=w322, "z phase"=w321, "calls per sample"="calls per sample (vel)", "index criteria"=w266, "active states"=w265) -> ("encoder position"=w320:i32, "velocity"=w313:i16)  [unwired: 5 in, 2 out]
    n159 = call-poly <vilib>:"nism.incremental.2.vi"("a phase"=w302, "reset"="Reset Encoder 2", "b phase"=w301, "z phase"=w300, "calls per sample"="calls per sample (vel)", "index criteria"=w266, "active states"=w265) -> ("encoder position"=w319:i32, "velocity"=w312:i16)  [unwired: 5 in, 2 out]
    n160 = call-poly <vilib>:"nism.incremental.2.vi"("a phase"=w293, "reset"="Reset Encoder 3", "b phase"=w292, "z phase"=w291, "calls per sample"="calls per sample (vel)", "index criteria"=w266, "active states"=w265) -> ("encoder position"=w318:i32, "velocity"=w311:i16)  [unwired: 5 in, 2 out]
    n161 = call-poly <vilib>:"nism.incremental.2.vi"("a phase"=w290, "reset"="Reset Encoder 4", "b phase"=w289, "z phase"=w288, "calls per sample"="calls per sample (vel)", "index criteria"=w266, "active states"=w265) -> ("encoder position"=w317:i32, "velocity"=w310:i16)  [unwired: 5 in, 2 out]
    n162 = call-poly <vilib>:"nism.incremental.2.vi"("a phase"=w277, "reset"="Reset Encoder 5", "b phase"=w276, "z phase"=w275, "calls per sample"="calls per sample (vel)", "index criteria"=w266, "active states"=w265) -> ("encoder position"=w316:i32, "velocity"=w309:i16)  [unwired: 5 in, 2 out]
    n163 = call-poly <vilib>:"nism.incremental.2.vi"("a phase"=w272, "reset"="Reset Encoder 6", "b phase"=w271, "z phase"=w270, "calls per sample"="calls per sample (vel)", "index criteria"=w266, "active states"=w265) -> ("encoder position"=w269:i32, "velocity"=w268:i16)  [unwired: 5 in, 2 out]
    n164 = Build Array(w320, w319, w318, w317, w316, w269) -> (w315:i32[])
    n165 = Build Array(w313, w312, w311, w310, w309, w268) -> (w314:i16[])
    n166 = global write "Global FPGA 6-axis.vi" "Unfiltered Position Feedback"(w315) -> ()
    n167 = global write "Global FPGA 6-axis.vi" "Unfiltered Velocity Feedback"(w314) -> ()
  }
  n168 = timed-loop "Synchronization Loop" {
    timing: w6 -> [_]
    timing-out: [_] -> w5
    stop <- FALSE stop-if-true
    n169 = xnode "FPGA I/O Node"() -> ("Scan Clock"=w336:bool)  [unwired: 1 in, 1 out]
    n170 = global read "Global FPGA 6-axis.vi" "Sync Enable"() -> (w335:bool)
    n171 = Select(t="Sync Value", s="Sync Enable override?", f=w335) -> (s? t:f=w332:bool)
    n172 = call-poly <vilib>:"nism.scan.generateSyncScan.vi"("scan enable?"=w332, "scan clock"=w336) -> ("timer control"=w337:T15)  [unwired: 3 in]
    n173 = global write "Global FPGA 6-axis.vi" "Timer Control"(w337) -> ()
  }
  n174 = timed-loop "Reset Monitoring Loop" {
    timing: w4 -> [_]
    timing-out: [_] -> w3
    stop <- FALSE stop-if-true
    n175 = global read "Global FPGA 6-axis.vi" "Reset Pending"() -> (w343:bool[])
    n176 = xnode "FPGA I/O Node"() -> ("Scan Clock"=w342:bool)  [unwired: 1 in, 1 out]
    n177 = feedback-in #1(w342) -> ()
    n178 = feedback #1() -> (w341:bool)  [unwired: 1 in]
    n179 = Greater?(x=w342, y=w341) -> (0:w347:bool)
    n180 = feedback #2() -> (w346:bool[])  [unwired: 1 in]
    n181 = Select(t=w343, s=w347, f=w346) -> (s? t:f=w344:bool[])
    n182 = feedback-in #2(w344) -> ()
    n183 = global write "Global FPGA 6-axis.vi" "Reset"(w344) -> ()
  }
  n184 = node-c288(w3) -> ()
  n185 = node-c288(w5) -> ()
  n186 = node-c288(w1) -> ()
